vi "Do Request.vi"(7 "Processing In":refnum<class "Processing.lvclass">, 11 "Pending Submissions in":refnum<class "Admin Info.lvclass">) -> (0 "error out":errorcluster, 5 "Processing":refnum<class "Processing.lvclass">)   [LabVIEW 2020, in "Summer of LabVIEW.lvlib" / "Admin Info.lvclass"]
uses:
  Admin Info.lvclass
  <vilib>/IlluminatedG/IG HTTP Server/HTTP Server/Processing/Processing.lvclass
  Submission DB/Submission DB.lvclass
  <vilib>/IlluminatedG/IG HTTP Server/HTTP Server/Security/Security.lvclass
  <vilib>/IlluminatedG/IG HTTP Server/HTTP Server/Processing/Processing.lvclass/Processing.ctl
  187530a3-3456-4252-bbf4-795405bb432f.vi
  57a7b61f-6e32-4309-806e-367723175dfc.vi
  187530a3-3456-4252-bbf4-795405bb432f.vi/9528e9df-aefc-4ce0-9221-106a337fd3b6.vi
  57a7b61f-6e32-4309-806e-367723175dfc.vi/9528e9df-aefc-4ce0-9221-106a337fd3b6.vi
  <vilib>/IlluminatedG/IG HTTP Server/HTTP Server/Values/Get Arg Map.vi
  <vilib>/Utility/error.llb/Error Cluster From Error Code.vi
  Admin Info.lvclass/Admin Info.ctl
  <vilib>/IlluminatedG/IG HTTP Utils/HTTP Utils/Response/Response.lvclass
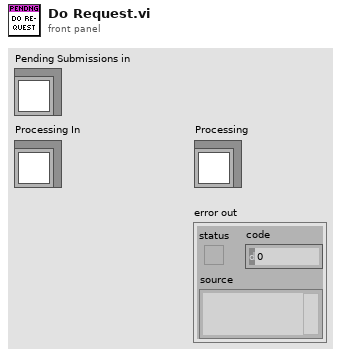
[diagram p1: front panel]
types:
  T1 = typedef "Summer of LabVIEW.lvlib/Admin Info JSON.ctl" = cluster{"Pending":T2[], "Running":T2[], "Completed":T2[]}
  T2 = typedef "Summer of LabVIEW.lvlib/Pending Submission JSON.ctl" = cluster{"sub_id":i64, "user_id":i64, "chal_id":i64, "submitted":string, "first_name":string, "last_name":string, "email":string, "department":string, "challenge":string, "score":dbl}
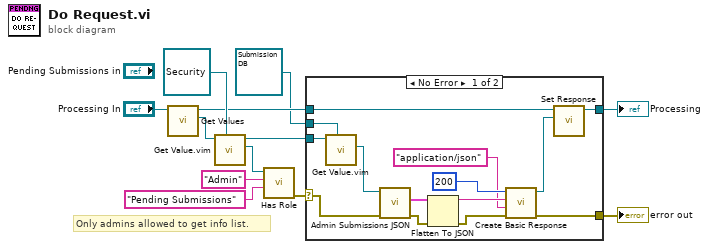
[diagram p0: block diagram]
diagram:
  # "Only admins allowed to get info list."
  n1 = call <vilib>:"Get Values.vi"("Processing in"="Processing In") -> ("Values"=w9:refnum<class "Values.lvclass">, "Processing out"=w3:refnum<class "Processing.lvclass">)  [unwired: 9 in]
  n2 = call "Get Value.vim"("Type / Server / Service (String)"=refnum<class "Security.lvclass"> refnum ("HTTP Server.lvlib:Security.lvclass"), "Arguments in"=w9) -> ("Value"=w7:refnum<class "Security.lvclass">, "Arguments out"=w2:refnum<class "Values.lvclass">)  [unwired: 7 in, 1 out]
  n3 = call <vilib>:"Has Role.vi"("Description (None)"="Pending Submissions" ("Role"), "Role"="Admin", "Security in"=w7) -> ("error out"=w4:errorcluster)  [unwired: 6 in, 2 out]
  n4 = case shown="No Error" w4 {
    selector: w4 -> [w17 w27]
    tunnel: [w19 w27] -> w12
    tunnel: [w18 w28] -> w11
    tunnel: w3 -> [w16 w28]
    tunnel: w2 -> [w15 _]
    tunnel: refnum<class "Submission DB.lvclass"> refnum ("SOL:Submission DB.lvclass") -> [w14 _]
    frame No Error {
      n5 = call "Get Value.vim"("Type / Server / Service (String)"=w14, "Arguments in"=w15) -> ("Value"=w13:refnum<class "Submission DB.lvclass">)  [unwired: 7 in, 2 out]
      n6 = call "Admin Submissions JSON.vi"("error in (no error)"=w17, "Submission DB in"=w13) -> ("error out"=w24:errorcluster, "Admin Info JSON"=w25:T1)  [unwired: 7 in, 1 out]
      n7 = Flatten To JSON(anything=w25, error in (no error)=w24) -> (JSON string=w23:string, 11:w26:errorcluster)  [unwired: 1 in]
      n8 = call <vilib>:"Create Basic Response.vi"("error in (no error)"=w26, "Content-Type (text/plain)"="application/json", "Payload"=w23, "Status Code"=u16 200) -> ("error out"=w19:errorcluster, "Response out"=w20:refnum<class "Response.lvclass">)  [unwired: 6 in]
      n9 = call <vilib>:"Set Response.vi"("Response"=w20, "Processing in"=w16) -> ("Processing out"=w18:refnum<class "Processing.lvclass">)  [unwired: 9 in]
    }
    frame Error {
    }
  }
  "error out" <- w12
  "Processing" <- w11
